vi "read_sensors.vi"(7 "baud rate":u32=9600, 8 "error in":errorcluster, 11 "VISA COM":refnum<visa-resource-name>) -> (0 "error out":errorcluster, 2 "sensor array":dbl[](array[numeric]), 3 "VISA COM":refnum<visa-resource-name>)   [LabVIEW 2018]
uses:
  <vilib>/Instr/_visa.llb/VISA Configure Serial Port (Instr).vi
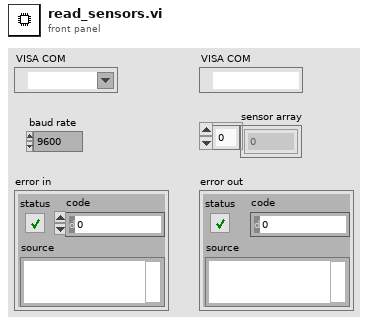
[diagram p1: front panel]
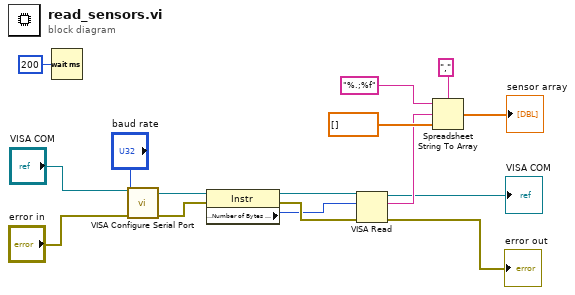
[diagram p0: block diagram]
diagram:
  n1 = Wait (ms)(milliseconds to wait=u32 200) -> ()  [unwired: 1 out]
  n2 = call-poly "VISA Configure Serial Port"("VISA resource name"="VISA COM", "baud rate (9600)"="baud rate", "error in (no error)"="error in") -> ("VISA resource name out"=w3:refnum<visa-resource-name>, "error out"=w4:errorcluster)  [unwired: 11 in]
  n3 = property class="Instr"(reference=w3, error in=w4) -> (reference out=w9:refnum<visa-resource-name>, error out=w10:errorcluster, "Serial Settings:Number of Bytes at Serial Port"=w8:u32)
  n4 = VISA Read(VISA resource name=w9, byte count=w8, error in (no error)=w10) -> (VISA resource name out=→"VISA COM":refnum<visa-resource-name>, read buffer=w12:string, error out=→"error out":errorcluster)  [unwired: 1 out]
  n5 = Spreadsheet String To Array(delimiter (Tab)=",", format string="%.;%f", spreadsheet string=w12, array type (2D Dbl)=dbl[] []) -> (array=→"sensor array":dbl[])
